vi "PADE (SubVI).vi"(9 "RETARDO":dbl, 10 "DENOMIDADOR":dbl[](array[numeric]), 11 "NUMERADOR":dbl[](array[numeric])) -> (2 "DENOMIDADOR  PADE":dbl[](array[numeric]), 3 "NUMERADOR  PADE":dbl[](array[numeric]))   [LabVIEW 2020]
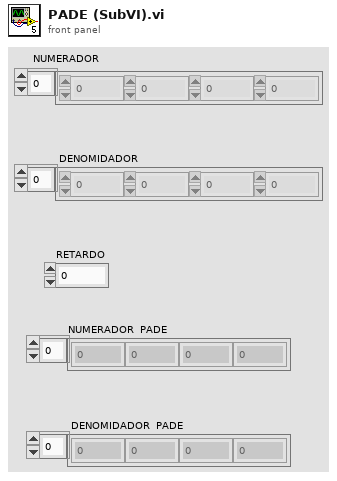
[diagram p1: front panel]
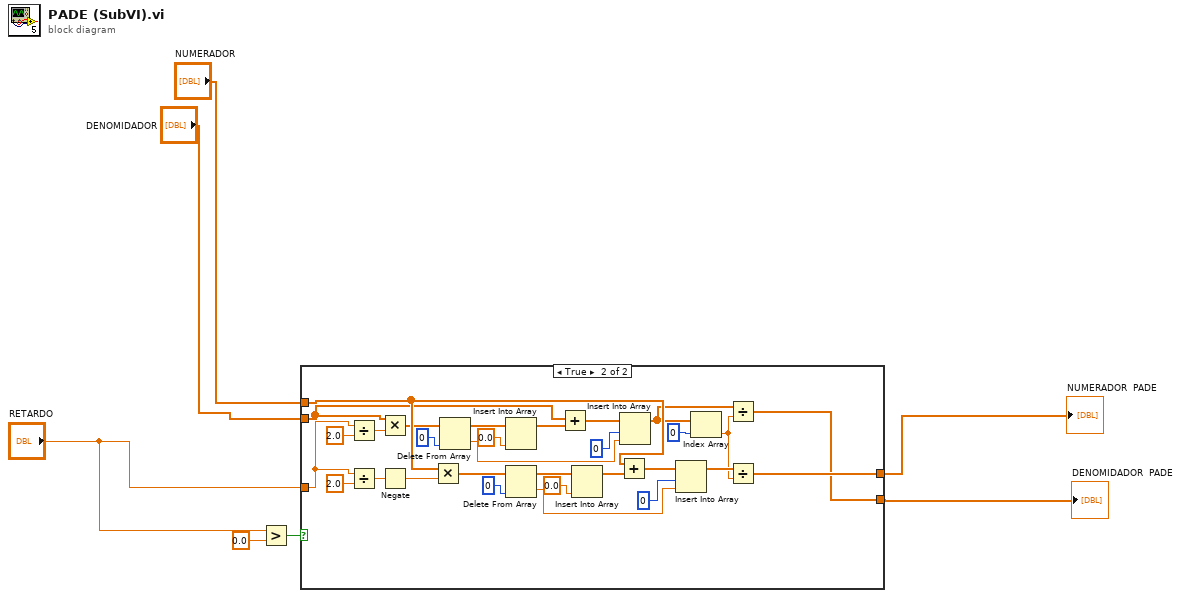
[diagram p0: block diagram]
diagram:
  n1 = Greater?(x="RETARDO", y=0.0) -> (0:w1:bool)
  n2 = case shown="True" w1 {
    tunnel: "NUMERADOR" -> [w9 w27]
    tunnel: "DENOMIDADOR" -> [w8 w14]
    tunnel: "RETARDO" -> [_ w13]
    tunnel: [w9 w11] -> w6
    tunnel: [w8 w10] -> w7
    frame False {
    }
    frame True {
      n3 = Divide(x=w13, y=2.0) -> (x/y=w17:dbl)
      n4 = Divide(x=w13, y=2.0) -> (x/y=w29:dbl)
      n5 = Multiply(x=w14, y=w17) -> (x*y=w20:dbl[])
      n6 = Negate(x=w29) -> (-x=w37:dbl)
      n7 = Multiply(x=w27, y=w37) -> (x*y=w36:dbl[])
      n8 = Delete From Array(array=w20, index=0) -> (deleted portion=w21:dbl, array with subset deleted=w23:dbl[])  [unwired: 1 in]
      n9 = Insert Into Array(array=w23, new element=0.0 ("new element/subarray")) -> (w26:dbl[])  [unwired: 1 in]
      n10 = Delete From Array(array=w36, index=0) -> (deleted portion=w35:dbl, array with subset deleted=w33:dbl[])  [unwired: 1 in]
      n11 = Add(x=w14, y=w26) -> (x+y=w22:dbl[])
      n12 = Insert Into Array(array=w33, new element=0.0 ("new element/subarray")) -> (w30:dbl[])  [unwired: 1 in]
      n13 = Add(x=w27, y=w30) -> (x+y=w34:dbl[])
      n14 = Insert Into Array(array=w22, index=0, new element=w21) -> (w16:dbl[])
      n15 = Insert Into Array(array=w34, index=0, new element=w35) -> (w28:dbl[])
      n16 = Index Array(array=w16, index=0) -> (element=w12:dbl)
      n17 = Divide(x=w16, y=w12) -> (x/y=w10:dbl[])
      n18 = Divide(x=w28, y=w12) -> (x/y=w11:dbl[])
    }
  }
  "DENOMIDADOR  PADE" <- w7
  "NUMERADOR  PADE" <- w6
